vi "FromRepo.vi"(8 "error in":errorcluster, 9 "from repo cluster":T2, 10 "repository in":refnum<class "NISE_CEF_Repository.lvclass">, 11 "node in":refnum<class "NISE_CEF_serializable node.lvclass">) -> (0 "error out":errorcluster, 2 "repository out":refnum<class "NISE_CEF_Repository.lvclass">, 3 "node":T1)   [LabVIEW 2013, in "NISE_CEF_serializable node.lvclass"]
doc: "Grabs information from the Repo and stores it in the nodes."
uses:
  NISE_CEF_serializable node.lvclass
  Repository/NISE_CEF_Repository.lvclass
  Node/FromRepoCluster.ctl
  Node/NodeRef.ctl
  Node/NISE_CEF_Node.lvclass
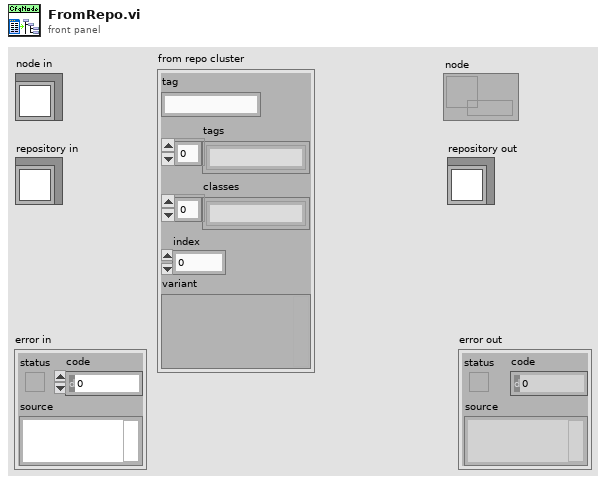
[diagram p1: front panel]
types:
  T1 = typedef "NISE_CEF_Node.lvclass/NodeRef.ctl" = refnum<data-value>
  T2 = typedef "NISE_CEF_Node.lvclass/FromRepoCluster.ctl" = cluster{"tag":string, "tags":string[], "classes":string[], "index":i32, "variant":variant}
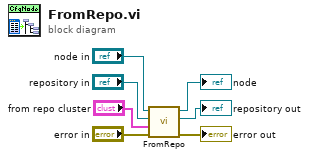
[diagram p0: block diagram]
diagram:
  n1 = call-parent "FromRepo.vi"("error in"="error in", "from repo cluster"="from repo cluster", "repository in"="repository in", "node in"="node in") -> ("error out"=→"error out":errorcluster, "repository out"=→"repository out":refnum<class "NISE_CEF_Repository.lvclass">, "node"=→"node":T1)  [unwired: 5 in]
